vi "Drive Code.vi"(0 "X Axis Input":dbl, 5 "Y Axis Input":dbl, 7 "Shift":bool, 9 "Manual Shooter":bool, 11 "Toggle Robot Reverse":bool) -> ()   [LabVIEW 2016]
uses:
  <vilib>/Rock Robotics/WPI/Solenoid/WPI_SolenoidValue.ctl
  <vilib>/Rock Robotics/WPI/Utilities/WPI_GetSetVariantRefNum.vi
  <vilib>/Rock Robotics/Network Tables/NT Write Numeric Array.vi
  <vilib>/Rock Robotics/Network Tables/NT Write Boolean Array.vi
  Robot Global Data.vi
  <vilib>/Rock Robotics/WPI/Solenoid/WPI_SolenoidSetEnum.vi
  <vilib>/addons/control/pid/pid.llb/PID (DBL).vi
  <vilib>/Rock Robotics/Network Tables/NT Write Number.vi
  <vilib>/addons/control/pid/NI_PID_pid.lvlib
panel:
  in  "Yaw Offset":dbl
  in  "PID gains":T1={"proportional gain (Kc)"=1.0, "integral time (Ti, min)"=0.01, "derivative time (Td, min)"=0.0} {"derivative time (Td, min)" format="%.3f"; "integral time (Ti, min)" format="%.3f"; "proportional gain (Kc)" format="%.3f"}
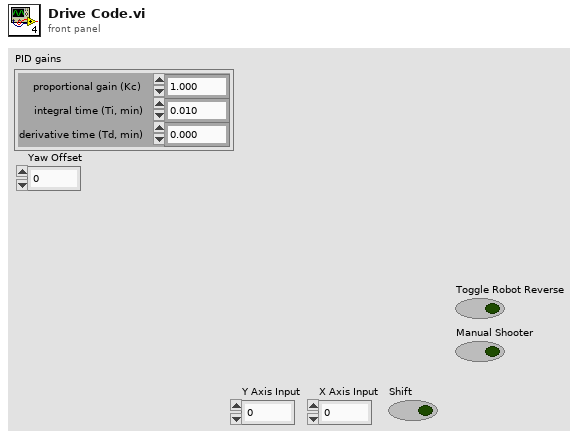
[diagram p1: front panel]
types:
  T1 = cluster{"proportional gain (Kc)":dbl, "integral time (Ti, min)":dbl, "derivative time (Td, min)":dbl}
  T2 = typedef "WPI_SolenoidValue.ctl" = enum16{"Off", "On", "Forward", "Reverse"}
  T3 = typedef "WPI_RobotDriveDevRef.ctl" = cluster{"DevStatus":errorcluster, "Motors[]":T4[], "Square Inputs":bool, "Max Output":dbl}
  T4 = typedef "WPI_MotorControlDeviceRef.ctl" = cluster{"DeviceStatus":errorcluster, "Type":T5, "PWM":cluster{"PWM Channel":T6, "DeadBand":T7}, "CAN":cluster{"Device Number":u8, "SetOutput VI Ref":variant, "GetOutput VI Ref":variant, "Enable VI Ref":variant, "Disable VI Ref":variant, "Data":variant}, "Invert":bool}
  T5 = typedef "WPI_MotorControlType.ctl" = enum16{"PWM", "CAN"}
  T6 = typedef "FPGA_DIOPWMChannel.ctl" = enum8{"PWM 0", "PWM 1", "PWM 2", "PWM 3", "PWM 4", "PWM 5", "PWM 6", "PWM 7", "PWM 8", "PWM 9", "PWM MXP 0", "PWM MXP 1", "PWM MXP 2", "PWM MXP 3", "PWM MXP 4", "PWM MXP 5", "PWM MXP 6", "PWM MXP 7", "PWM MXP 8", "PWM MXP 9", "Invalid"}
  T7 = typedef "WPI_PWMDeadband.ctl" = cluster{"Name":string, "maxPositivePwm":i32, "minPositivePwm":i32, "centerPwm":i32, "maxNegativePwm":i32, "minNegativePwm":i32, "angularRange":u16}
  T8 = typedef "WPI_JoystickDevRef.ctl" = cluster{"Device":T9}
  T9 = typedef "WPI_JoystickDeviceEnum.ctl" = enum16{"USB 0", "USB 1", "USB 2", "USB 3", "USB 4", "USB 5"}
  T10 = typedef "WPI_DigitalInputDevRef.ctl" = cluster{"DevStatus":errorcluster, "DIO Channel":T11}
  T11 = typedef "FPGA_DIOChannel.ctl" = enum8{"DIO 0", "DIO 1", "DIO 2", "DIO 3", "DIO 4", "DIO 5", "DIO 6", "DIO 7", "DIO 8", "DIO 9", "DIO MXP 0", "DIO MXP 1", "DIO MXP 2", "DIO MXP 3", "DIO MXP 4", "DIO MXP 5", "DIO MXP 6", "DIO MXP 7", "DIO MXP 8", "DIO MXP 9", "DIO MXP 10", "DIO MXP 11", "DIO MXP 12", "DIO MXP 13", "DIO MXP 14", "DIO MXP 15", "SPI Port CS1", "SPI Port CS2", "SPI Port CS3", "SPI Port MISO", "SPI Port MOSI", "Invalid"}
  T12 = typedef "WPI_AnalogChannelDevRef.ctl" = cluster{"DevStatus":errorcluster, "Analog Channel":T13}
  T13 = typedef "FPGA_AIChannel.ctl" = enum8{"AI 0", "AI 1", "AI 2", "AI 3", "AI MXP 0", "AI MXP 1", "AI MXP 2", "AI MXP 3", "Invalid"}
  T14 = typedef "WPI_SolenoidDevRef.ctl" = cluster{"DevStatus":errorcluster, "Pneumatics Control Module":u8, "Forward Solenoid Channel":T15, "Reverse Solenoid Channel":T15}
  T15 = typedef "WPI_SolenoidChannel.ctl" = enum8{"Solenoid 0", "Solenoid 1", "Solenoid 2", "Solenoid 3", "Solenoid 4", "Solenoid 5", "Solenoid 6", "Solenoid 7", "Invalid"}
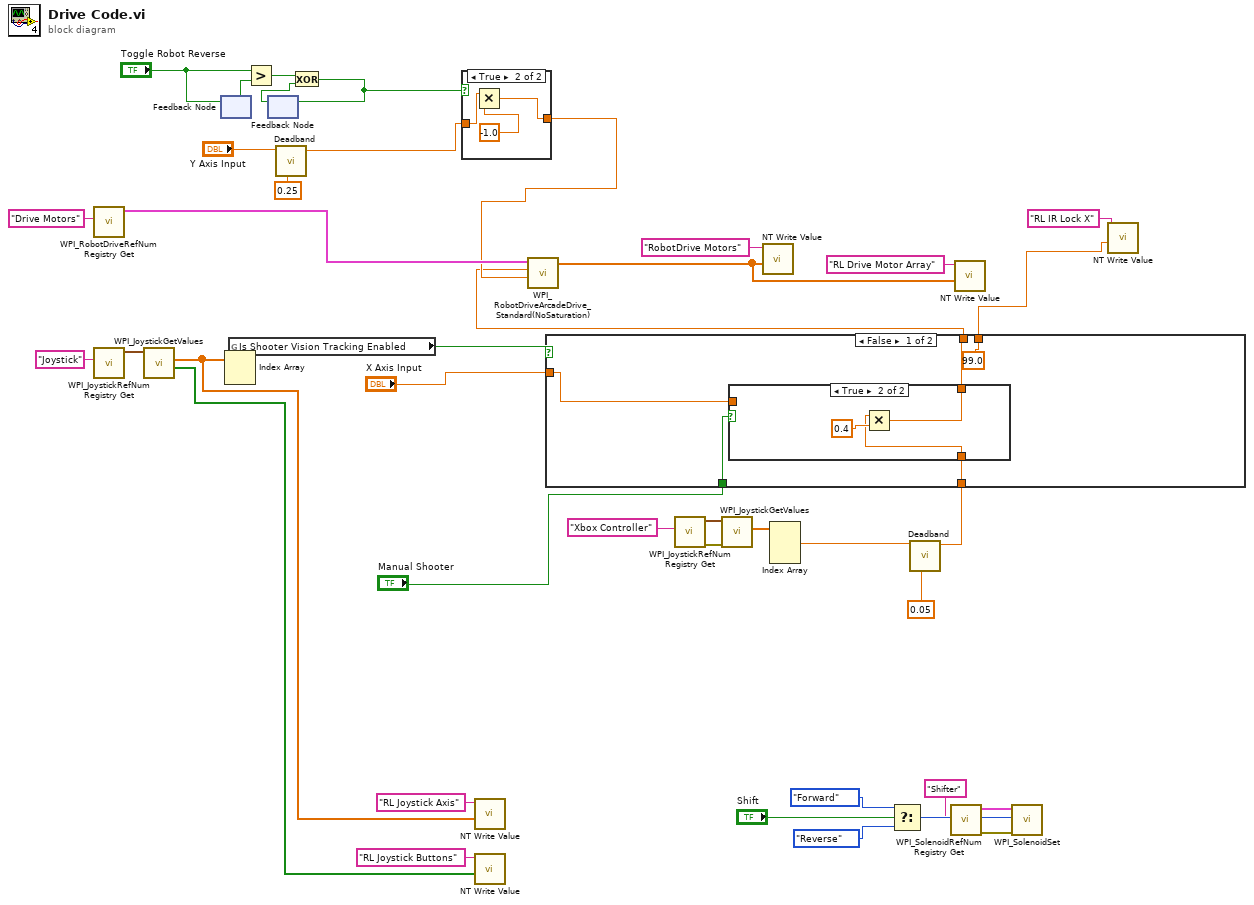
[diagram p0: block diagram]
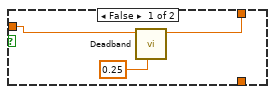
[diagram p3: hidden frame]
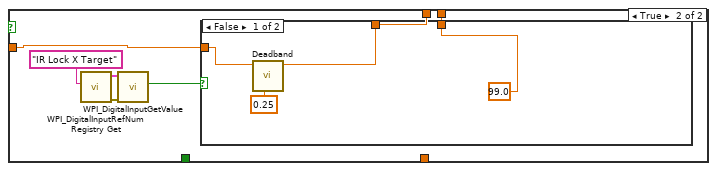
[diagram p4: hidden frame]
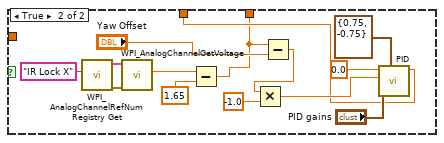
[diagram p5: hidden frame]
diagram:
  n1 = call <vilib>:"WPI_RobotDriveRefNum Registry Get.vi"("refnum name"="Drive Motors") -> ("RobotDriveDevRef"=w40:T3)  [unwired: 1 in, 9 out]
  n2 = call <vilib>:"WPI_JoystickRefNum Registry Get.vi"("refnum name"="Joystick") -> ("JoystickDevRef"=w39:T8)  [unwired: 1 in, 9 out]
  n3 = call <vilib>:"WPI_JoystickGetValues.vi"("JoystickDevRef"=w39) -> ("Buttons"=w10:bool[], "Axes"=w35:dbl[])  [unwired: 6 in, 3 out]
  n4 = feedback-in #1("Toggle Robot Reverse") -> ()
  n5 = feedback #1() -> (w20:bool)  [unwired: 1 in]
  n6 = Index Array(array=w35) -> ()  [unwired: 2 in, 2 out]
  n7 = global read "Robot Global Data.vi" "Is Shooter Vision Tracking Enabled"() -> (w23:bool)
  n8 = Greater?(x="Toggle Robot Reverse", y=w20) -> (0:w21:bool)
  n9 = feedback #2() -> (w19:bool)  [unwired: 1 in]
  n10 = call "Deadband.vi"("Value"=0.25, "Input"="Y Axis Input") -> ("Output"=w22:dbl)  [unwired: 9 in]
  n11 = Exclusive Or(1:w19, 2:w21) -> (0:w18:bool)
  n12 = feedback-in #2(w18) -> ()
  n13 = case shown="True" w18 {
    tunnel: w22 -> [w41 w44]
    tunnel: [w41 w42] -> w17
    frame False {
    }
    frame True {
      n14 = Multiply(x=w44, y=-1.0) -> (x*y=w42:dbl)
    }
  }
  n15 = call-poly <vilib>:"NT Write Value.vi"("Numeric Array"=w35, "Name"="RL Joystick Axis") -> ()  [unwired: 9 in, 1 out]
  n16 = call-poly <vilib>:"NT Write Value.vi"("Boolean Array"=w10, "Name"="RL Joystick Buttons") -> ()  [unwired: 9 in, 1 out]
  n17 = call <vilib>:"WPI_JoystickRefNum Registry Get.vi"("refnum name"="Xbox Controller") -> ("error out"=w13:errorcluster, "JoystickDevRef"=w14:T8)  [unwired: 1 in, 8 out]
  n18 = call <vilib>:"WPI_JoystickGetValues.vi"("error in (no error)"=w13, "JoystickDevRef"=w14) -> ("Axes"=w12:dbl[])  [unwired: 5 in, 4 out]
  n19 = Index Array(array=w12) -> (element #1=w8:dbl)  [unwired: 3 in, 2 out]
  n20 = Select(t=WPI_SolenoidValue."Forward" ("Value"), s="Shift", f=WPI_SolenoidValue."Reverse" ("Value")) -> (s? t:f=w29:T2)
  n21 = call "Deadband.vi"("Value"=0.05, "Input"=w8) -> ("Output"=w9:dbl)  [unwired: 9 in]
  n22 = case shown="False" w23 {
    tunnel: [w46 w57] -> w16
    tunnel: "X Axis Input" -> [w48 w58]
    tunnel: "Manual Shooter" -> [w49 _]
    tunnel: w9 -> [w47 _]
    tunnel: [99.0 w56] -> w1
    frame False {
      n23 = case shown="True" w49 {
        tunnel: w48 -> [w51 _]
        tunnel: w47 -> [_ w54]
        tunnel: [w50 w53] -> w46
        frame False {
          n24 = call "Deadband.vi"("Value"=0.25, "Input"=w51) -> ("Output"=w50:dbl)  [unwired: 9 in]
        }
        frame True {
          n25 = Multiply(x=w54, y=0.4) -> (x*y=w53:dbl)
        }
      }
    }
    frame True {
      n26 = call <vilib>:"WPI_DigitalInputRefNum Registry Get.vi"("refnum name"="IR Lock X Target") -> ("error out"=w61:errorcluster, "DigitalInputDevRef"=w62:T10)  [unwired: 9 in]
      n27 = call <vilib>:"WPI_DigitalInputGetValue.vi"("error in (no error)"=w61, "DigitalInputDevRef"=w62) -> ("Value"=w59:bool)  [unwired: 7 in, 2 out]
      n28 = case shown="False" w59 {
        tunnel: w58 -> [w65 _]
        tunnel: [w64 w70] -> w57
        tunnel: [99.0 w67] -> w56
        frame False {
          n29 = call "Deadband.vi"("Value"=0.25, "Input"=w65) -> ("Output"=w64:dbl)  [unwired: 9 in]
        }
        frame True {
          n30 = call <vilib>:"WPI_AnalogChannelRefNum Registry Get.vi"("refnum name"="IR Lock X") -> ("error out"=w77:errorcluster, "AIDeviceRef"=w78:T12)  [unwired: 9 in]
          n31 = call <vilib>:"WPI_AnalogChannelGetVoltage.vi"("error in (no error)"=w77, "AIDeviceRef"=w78) -> ("Voltage"=w80:dbl)  [unwired: 7 in, 2 out]
          n32 = Subtract(x=w80, y=1.65) -> (x-y=w67:dbl)
          n33 = Subtract(x=w67, y="Yaw Offset") -> (x-y=w69:dbl)
          n34 = Multiply(x=w69, y=-1.0) -> (x*y=w73:dbl)
          n35 = call-poly <vilib>:"PID.vi"("output range"=cluster{"output high":dbl, "output low":dbl} {"output high"=0.75, "output low"=-0.75}, "PID gains"="PID gains", "process variable"=w73, "setpoint"=0.0) -> ("output"=w70:dbl)  [unwired: 6 in, 1 out]
        }
      }
    }
  }
  n36 = call <vilib>:"WPI_RobotDriveArcadeDrive_Standard(NoSaturation).vi"("Y axis value"=w17, "X axis value"=w16, "RobotDriveDevRef"=w40) -> ("Motor Values"=w33:dbl[])  [unwired: 1 in, 7 out]
  n37 = call-poly <vilib>:"NT Write Value.vi"("Numeric Array"=w33, "Name"="RobotDrive Motors") -> ()  [unwired: 9 in, 1 out]
  n38 = call <vilib>:"WPI_SolenoidRefNum Registry Get.vi"("refnum name"="Shifter") -> ("error out"=w30:errorcluster, "SolenoidDevRef"=w31:T14)  [unwired: 9 in]
  n39 = call-poly <vilib>:"NT Write Value.vi"("Numeric Array"=w33, "Name"="RL Drive Motor Array") -> ()  [unwired: 9 in, 1 out]
  n40 = call-poly <vilib>:"WPI_SolenoidSet.vi"("error in (no error)"=w30, "Value"=w29, "SolenoidDevRef"=w31) -> ()  [unwired: 7 in, 2 out]
  n41 = call-poly <vilib>:"NT Write Value.vi"("Numeric"=w1, "Name"="RL IR Lock X") -> ()  [unwired: 9 in, 1 out]
